vi "COM Descriptor Demo.vi"() -> ()   [LabVIEW 2020, in "Get COM Descriptor.lvlib"]
doc: "Get COM descriptor test panel."
uses:
  Get COM Descriptor.lvlib
  COM port.ctl
panel:
  out "COM list":T1[](array[typedef])
  in  "btn rescan":bool
  out "DLL version info string":string
  in  "btn exit":bool
  out "COM port Descriptor":string
  in  "VISA resource name":refnum<visa-resource-name>
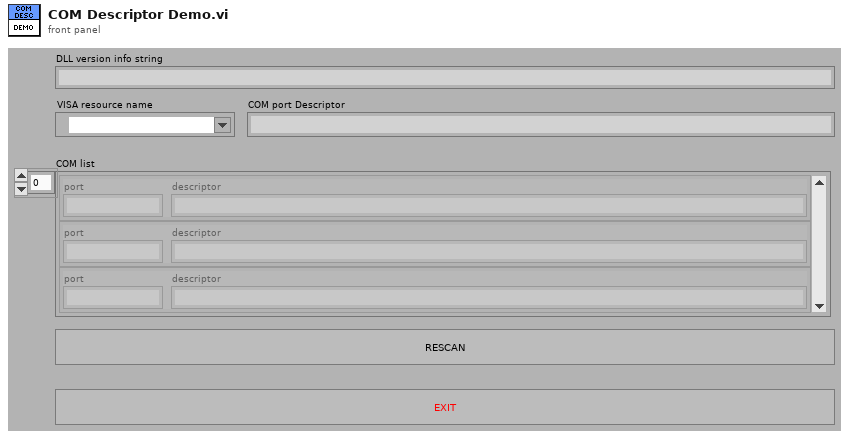
[diagram p1: front panel]
types:
  T1 = typedef "Get COM Descriptor.lvlib/COM port.ctl" = cluster{"port":string, "descriptor":string}
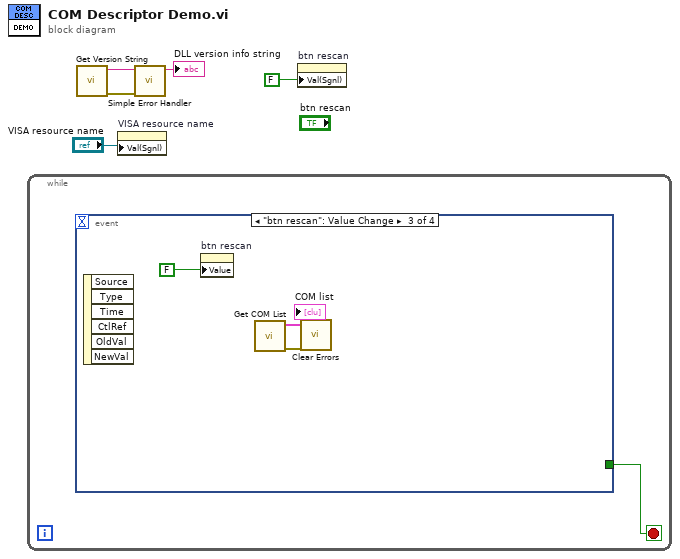
[diagram p0: block diagram]
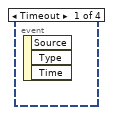
[diagram p2: hidden frame]
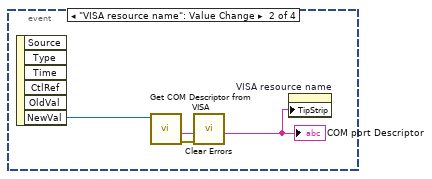
[diagram p3: hidden frame]
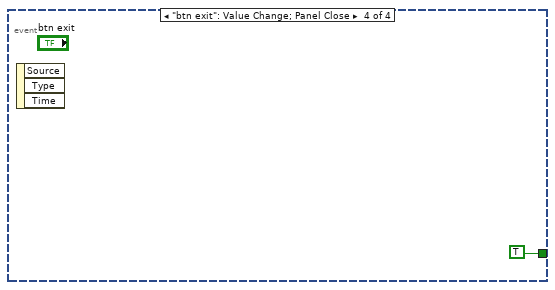
[diagram p4: hidden frame]
diagram:
  n1 = while {
    stop <- w5 stop-if-true
    n2 = event shown="[2] \"btn rescan\": Value Change" {
      selector: _ -> [_ _ _ _]
      dyn-events: _ -> [_ _ _ _]
      timeout: _ -> [_ _ _ _]
      tunnel: [_ _ _ TRUE] -> w5
      event Timeout {
        n3 = event-data() -> ()  [unwired: 1 in, 3 out]
      }
      event "VISA resource name": Value Change {
        n4 = event-data() -> ("NewVal"=w8:refnum<visa-resource-name>)  [unwired: 1 in, 5 out]
        n5 = call "Get COM Descriptor from VISA.vi"("VISA resource name"=w8) -> ("error out"=w7:errorcluster, "COM port Descriptor"=w6:string)  [unwired: 7 in, 2 out]
        "COM port Descriptor" <- w6
        n6 = call <vilib>:"Clear Errors.vi"("error in (no error)"=w7) -> ()  [unwired: 5 in, 2 out]
        n7 = property on="VISA resource name" class="VISAName"("TipStrip"=w6) -> ()  [unwired: 2 in, 2 out]
      }
      event "btn rescan": Value Change {
        n8 = event-data() -> ()  [unwired: 1 in, 6 out]
        n9 = property on="btn rescan" class="Bool (strict)"("Value"=FALSE) -> ()  [unwired: 2 in, 2 out]
        n10 = call "Get COM List.vi"() -> ("error out"=w11:errorcluster, "COM list"=→"COM list":T1[])  [unwired: 8 in, 2 out]
        n11 = call <vilib>:"Clear Errors.vi"("error in (no error)"=w11) -> ()  [unwired: 5 in, 2 out]
      }
      event "btn exit": Value Change; Panel Close {
        n12 = event-data() -> ()  [unwired: 1 in, 3 out]
      }
    }
  }
  n13 = call "Get Version String.vi"() -> ("error out"=w3:errorcluster, "version info string"=→"DLL version info string":string)  [unwired: 10 in]
  n14 = property on="VISA resource name" class="VISAName"("Val(Sgnl)"="VISA resource name") -> ()  [unwired: 2 in, 2 out]
  n15 = call <vilib>:"Simple Error Handler.vi"("error in (no error)"=w3) -> ()  [unwired: 4 in, 5 out]
  n16 = property on="btn rescan" class="Bool (strict)"("Val(Sgnl)"=FALSE) -> ()  [unwired: 2 in, 2 out]
